vi "Front Color Changed Action.vi"(8 "error in (no error)":errorcluster caption="错误输入（无错误）", 10 "Color":u32(colorbox), 11 "Control Ref":refnum<vi>[](array[refnum])) -> (0 "error out":errorcluster caption="错误输出")   [LabVIEW 2013, in "IP Adresss Control.xctl"]
uses:
  IP Adresss Control.xctl
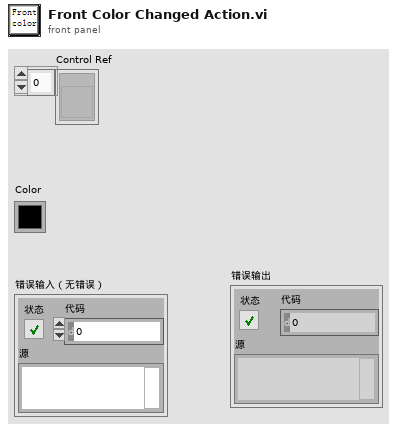
[diagram p1: front panel]
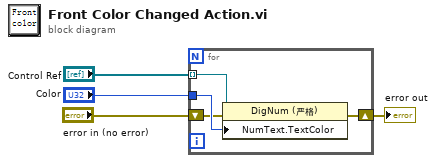
[diagram p0: block diagram]
diagram:
  n1 = for {
    tunnel: "Color" -> [w8]
    tunnel: "Control Ref" -> [w7] mode=indexing
    shift-right: [w6] -> w2
    shift-left: "error in (no error)" -> [w5]
    n2 = property class="DigNum (严格)"(reference=w7, error in=w5, "NumText.TextColor"=w8) -> (error out=w6:errorcluster)  [unwired: 1 out]
  }
  "error out" <- w2
